vi "LEBITplc.GetAddress.vi"(2 "channel# (dec)":i32, 3 "base Actual addr. (oct)":string) -> (0 "is a double?":bool, 1 "act. addr. (oct)":string)   [LabVIEW 2014, in "LEBITplc.lvlib"]
uses:
  LEBITplc.lvlib
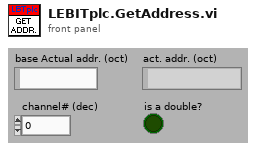
[diagram p1: front panel]
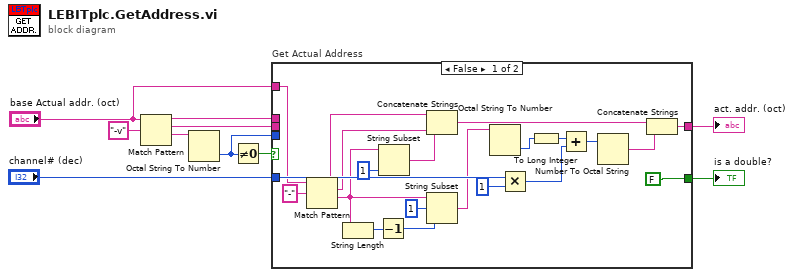
[diagram p0: block diagram]
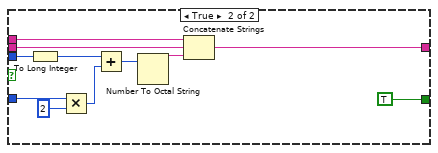
[diagram p2: hidden frame]
diagram:
  n1 = Match Pattern(string="base Actual addr. (oct)", regular expression="-v" ("search string")) -> (before substring=w3:string, match substring=w2:string, after substring=w6:string)  [unwired: 1 in, 1 out]
  n2 = Octal String To Number(4:w6) -> (0:w4:u32)  [unwired: 2 in, 1 out]
  n3 = Not Equal To 0?(x=w4) -> (x != 0?=w5:bool)
  n4 = case "Get Actual Address" shown="False" w5 {
    tunnel: "channel# (dec)" -> [w30 w40]
    tunnel: "base Actual addr. (oct)" -> [w18 _]
    tunnel: [w28 w38] -> w9
    tunnel: w4 -> [_ w33]
    tunnel: w3 -> [_ w37]
    tunnel: w2 -> [_ w36]
    tunnel: [FALSE TRUE] -> w1
    frame False {
      n5 = Match Pattern(string=w18, regular expression="-") -> (before substring=w23:string, match substring=w22:string, after substring=w21:string)  [unwired: 1 in, 1 out]
      n6 = String Length(string=w21) -> (length=w26:i32)
      n7 = Decrement(x=w26) -> (x-1=w24:i32)
      n8 = String Subset(string=w21, length (rest)=1 ("length (rest)")) -> (substring=w19:string)  [unwired: 1 in]
      n9 = Concatenate Strings(w23, w22, w19) -> (w17:string)
      n10 = String Subset(string=w21, offset (0)=1, length (rest)=w24) -> (substring=w16:string)
      n11 = Octal String To Number(4:w16) -> (0:w12:u32)  [unwired: 2 in, 1 out]
      n12 = Multiply(x=w30, y=1) -> (x*y=w14:i32)
      n13 = To Long Integer(number=w12) -> (32bit integer=w13:i32)
      n14 = Add(x=w13, y=w14) -> (x+y=w31:i32)
      n15 = Number To Octal String(2:w31) -> (0:w29:string)  [unwired: 1 in]
      n16 = Concatenate Strings(w17, w29) -> (w28:string)
    }
    frame True {
      n17 = To Long Integer(number=w33) -> (32bit integer=w34:i32)
      n18 = Multiply(x=w40, y=2) -> (x*y=w35:i32)
      n19 = Add(x=w34, y=w35) -> (x+y=w42:i32)
      n20 = Number To Octal String(2:w42) -> (0:w39:string)  [unwired: 1 in]
      n21 = Concatenate Strings(w37, w36, w39) -> (w38:string)
    }
  }
  "act. addr. (oct)" <- w9
  "is a double?" <- w1
